vi "Update Buffer.vi"(8 "Error in":errorcluster, 10 "Wfm data":dbl[][](array[numeric]), 11 "Async State Vars":T1) -> (0 "Error out":errorcluster, 3 "Async State Vars out":T1)   [LabVIEW 2014]
uses:
  Types/Async State Vars.ctl
  Types/Async FIFOs.ctl
  <vilib>/NI Veristand/Custom Device Waveform API/Single Waveform Read (DBL)/Single Waveform Read (DBL).lvclass
  <vilib>/NI Veristand/Custom Device Waveform API/Single Waveform Write (DBL)/Single Waveform Write (DBL).lvclass
  <vilib>/NI Veristand/Custom Device API/Waveform Data Reference.ctl
  <userlib>/Circular Buffer/Controls/Circular Buffer Operations.ctl
  <userlib>/Circular Buffer/Instance VIs/Circular Buffer(2D DBL).vi
  <userlib>/Circular Buffer/Circular Buffer.lvlib
  Waveform-Processing-Custom-Device Engine.lvlib
  <vilib>/NI Veristand/Custom Device API/Custom Device API.lvlib
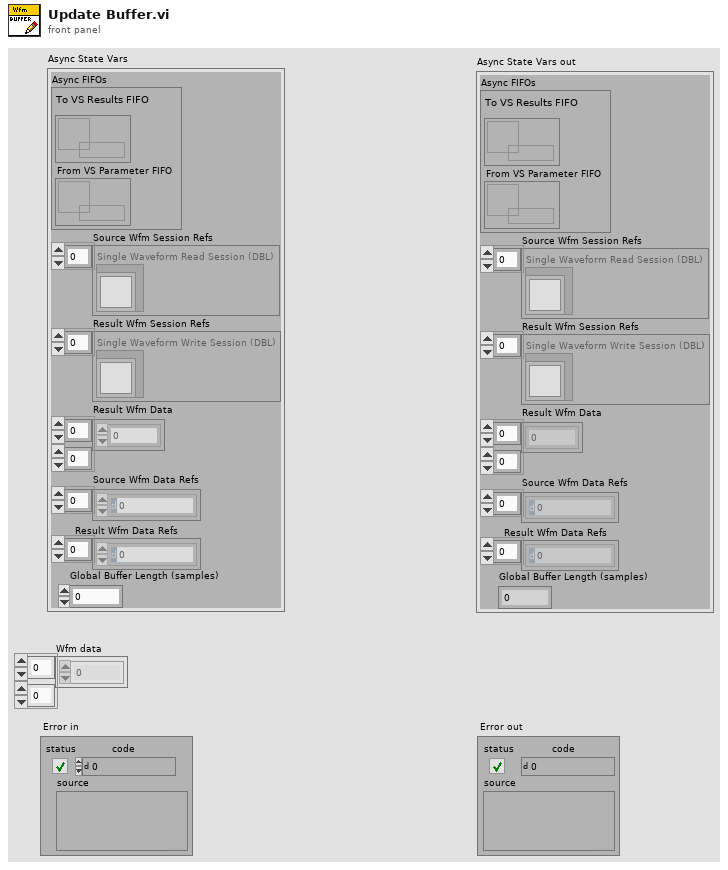
[diagram p1: front panel]
types:
  T1 = typedef "Waveform-Processing-Custom-Device Engine.lvlib/Async State Vars.ctl" = cluster{"Async FIFOs":T2, "Source Wfm Session Refs":refnum<class "Single Waveform Read (DBL).lvclass">[], "Result Wfm Session Refs":refnum<class "Single Waveform Write (DBL).lvclass">[], "Result Wfm Data":dbl[][], "Source Wfm Data Refs":T3[], "Result Wfm Data Refs":T3[], "Global Buffer Length (samples)":dbl}
  T2 = typedef "Waveform-Processing-Custom-Device Engine.lvlib/Async FIFOs.ctl" = cluster{"To VS Results FIFO":refnum<k33>, "From VS Parameter FIFO":refnum<k33>}
  T3 = typedef "Custom Device API.lvlib/Waveform Data Reference.ctl" = i32
  T4 = typedef "Circular Buffer.lvlib/Circular Buffer Operations.ctl" = enum16{"Initialize", "Get Backlog", "Write", "Read (continuous)", "Read (most recent)"}
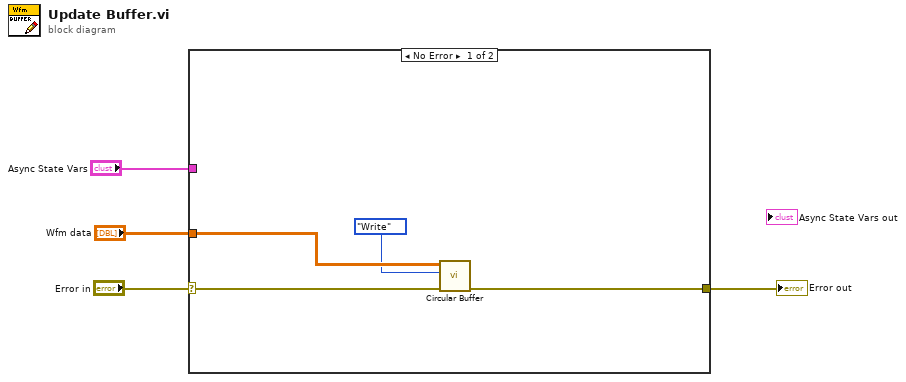
[diagram p0: block diagram]
diagram:
  n1 = case shown="No Error" "Error in" {
    selector: "Error in" -> [w8 w9]
    tunnel: [w7 w9] -> w3
    tunnel: "Wfm data" -> [w6 _]
    tunnel: "Async State Vars" -> [_ _]
    frame No Error {
      n2 = call-poly <userlib>:"Circular Buffer.vi"("error in (no error)"=w8, "Operation"=Circular_Buffer_Operations."Write", "Data In"=w6) -> ("error out"=w7:errorcluster)  [unwired: 5 in, 3 out]
    }
    frame Error {
    }
  }
  "Error out" <- w3
